vi "CANOpen_Main_Create and Send SDOs.vi"(7 "SDO Asynch":T1 {"HW Dyn Read"."Resp Chan."."Chan Refs" format="%.0x"; "HW Dyn Read"."Req Chan."."Chan Refs" format="%.0x"; "HW Dyn Write"."Resp Chan."."Chan Refs" format="%.0x"; "HW Dyn Write"."Req Chan."."Chan Refs" format="%.0x"; "List SDO"."Resp Chan."."Chan Refs" format="%.0x"; "List SDO"."Req Chan."."Chan Refs" format="%.0x"}, 8 "error in (no error)":errorcluster, 9 "Node States":u16[](array[ring]) items=["unknown"=1, "bootup"=0, "stopped"=4, "operational"=5, "pre-operational"=127, "connection lost"=128], 10 "Nodes":T3[](array[typedef]) {"NMT"."Node init static SDO state" items=["start remote node"=1, "enter pre-operational"=128]; "NMT"."Node run state" items=["start remote node"=1, "stop remote node"=2, "enter pre-operational"=128, "reset node"=129, "reset communication"=130]; "Dynamic SDOs"."Sub-Index (0)" format="%.0x"; "Dynamic SDOs"."Object Index" format="%.0x"; "Dynamic SDOs"."Block Data" format="%.0x"; "RPDOs"."PDO Channel" items=["PDO 1", "PDO 2", "PDO 3", "PDO 4"]; "RPDOs"."Parameters"."Bit Offset" max=8 step=1; "RPDOs"."Parameters"."Byte Offset" max=8 step=1; "TPDOs"."PDO Channel" items=["PDO 1", "PDO 2", "PDO 3", "PDO 4"]; "TPDOs"."Parameters"."Bit Offset" max=8 step=1; "TPDOs"."Parameters"."Byte Offset" max=8 step=1; "SDOs"."Sub-Index (0)" format="%.0x"; "SDOs"."Object Index" format="%.0x"; "SDOs"."Block Data" format="%.0x"}, 11 "interface object":refnum<k20>) -> (0 "error out":errorcluster, 3 "interface object out":refnum<k20>)   [LabVIEW 2013]
uses:
  SubVIS/CANOpen_Node Message Settings.ctl
  Shared Code/CANOpen_PDO Settings.ctl
  Shared Code/CANOpen_PDO Parameter Settings.ctl
  Shared Code/CANOpen_PDO Data Type.ctl
  System Explorer/SubVIs/CANopen Byte Order.ctl
  Shared Code/CANOpen_SDO Settings.ctl
  SubVIS/CANOpen_NMT Settings.ctl
  CanOpen_NMT_Config.ctl
  CanOpen_NMT_Static detect.ctl
  SubVIS/CANOpen_VS SDOs Data Refs.ctl
  <vilib>/NI Veristand/Custom Device API/Data Reference.ctl
  CanOpen_SDO Dynamic queue.ctl
  Shared Code/CANOpen_SDO queue W data.ctl
  Shared Code/CANOpen_SDO queue mode.ctl
  Shared Code/CANOpen_PDO Data Type in queue.ctl
  <vilib>/CANopenLib/CANOPEN.llb/CANopen SDO Create.vi
  <vilib>/CANopenLib/CANOPEN.llb/CANopen SDO Write [Block].vi
  <vilib>/CANopenLib/CANOPEN.llb/CANopen SDO Close.vi
  CANOpen Addon Custom Device.lvlib
  <vilib>/NI Veristand/Custom Device API/Custom Device API.lvlib
panel:
  # "LSB"
  # "MSB"
  # "LSB"
  # "MSB"
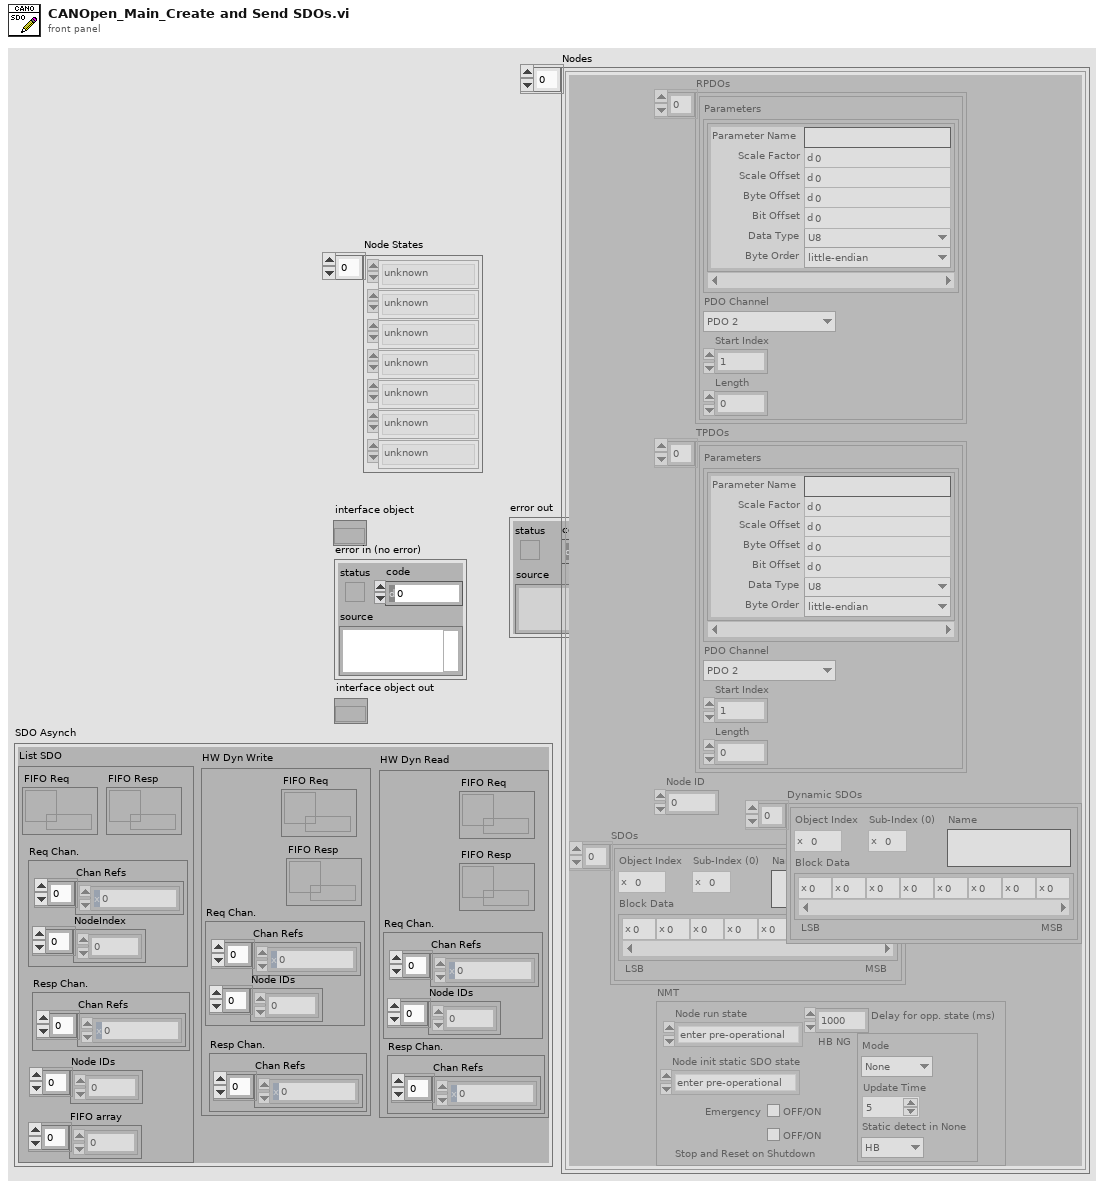
[diagram p1: front panel]
types:
  T1 = typedef "CANOpen Addon Custom Device.lvlib/CANOpen_VS SDOs Data Refs.ctl" = cluster{"List SDO":cluster{"FIFO Req":refnum<k33>, "Req Chan.":cluster{"Chan Refs":T2[], "NodeIndex":dbl[]}, "FIFO Resp":refnum<k33>, "Resp Chan.":cluster{"Chan Refs":T2[]}, "Node IDs":u8[], "FIFO array":dbl[]}, "HW Dyn Write":cluster{"FIFO Req":refnum<k33>, "FIFO Resp":refnum<k33>, "Req Chan.":cluster{"Chan Refs":T2[], "Node IDs":u8[]}, "Resp Chan.":cluster{"Chan Refs":T2[]}}, "HW Dyn Read":cluster{"FIFO Req":refnum<k33>, "FIFO Resp":refnum<k33>, "Req Chan.":cluster{"Chan Refs":T2[], "Node IDs":u8[]}, "Resp Chan.":cluster{"Chan Refs":T2[]}}}
  T2 = typedef "Custom Device API.lvlib/Data Reference.ctl" = i32
  T3 = typedef "CANOpen_Node Message Settings.ctl" = cluster{"RPDOs":T4[], "TPDOs":T4[], "Node ID":u8, "SDOs":T8[], "Dynamic SDOs":T8[], "NMT":T9}
  T4 = typedef "CANOpen Addon Custom Device.lvlib/CANOpen_PDO Settings.ctl" = cluster{"Parameters":T5[], "PDO Channel":u8, "Start Index":u32, "Length":u32}
  T5 = typedef "CANOpen Addon Custom Device.lvlib/CANOpen_PDO Parameter Settings.ctl" = cluster{"Parameter Name":string, "Scale Factor":dbl, "Scale Offset":dbl, "Byte Offset":u8, "Bit Offset":u8, "Data Type":T6, "Byte Order":T7}
  T6 = typedef "CANOpen Addon Custom Device.lvlib/CANOpen_PDO Data Type.ctl" = enum16{"U8", "U16", "U32", "I8", "I16", "I32", "Single", "Double", "Boolean"}
  T7 = typedef "CANOpen Addon Custom Device.lvlib/CANopen Byte Order.ctl" = enum16{"big-endian network order", "little-endian"}
  T8 = typedef "CANOpen Addon Custom Device.lvlib/CANOpen_SDO Settings.ctl" = cluster{"Object Index":u16, "Sub-Index (0)":u8, "Block Data":u8[], "Name":string}
  T9 = typedef "CANOpen Addon Custom Device.lvlib/CANOpen_NMT Settings.ctl" = cluster{"Node run state":u16, "Emergency":bool, "HB NG":T10, "Delay for opp. state (ms)":dbl, "Node init static SDO state":u16, "Stop and Reset on Shutdown":bool}
  T10 = typedef "CANOpen Addon Custom Device.lvlib/CanOpen_NMT_Config.ctl" = cluster{"Mode":T11, "Update Time":u16, "Static detect in None":T11}
  T11 = typedef "CANOpen Addon Custom Device.lvlib/CanOpen_NMT_Static detect.ctl" = enum16{"None", "HB", "NG"}
  T12 = typedef "CANOpen Addon Custom Device.lvlib/CANOpen_SDO queue mode.ctl" = enum16{"WRITE write", "WRITE response", "READ write", "READ response"}
  T13 = typedef "CANOpen Addon Custom Device.lvlib/CANOpen_PDO Data Type in queue.ctl" = enum16{"U8", "U16", "U32", "I8", "I16", "I32", "Single", "Double"}
  T14 = typedef "CANOpen Addon Custom Device.lvlib/CanOpen_SDO Dynamic queue.ctl" = cluster{"Node ID":u8, "Data":T15}
  T15 = typedef "CANOpen Addon Custom Device.lvlib/CANOpen_SDO queue W data.ctl" = cluster{"Object Index":u16, "Object Sub-Index (0)":u8, "Mode":T12, "Data Type":T13, "Value":dbl, "Status code":dbl, "Byte Order":enum16{"big-endian, network order", "little-endian"}}
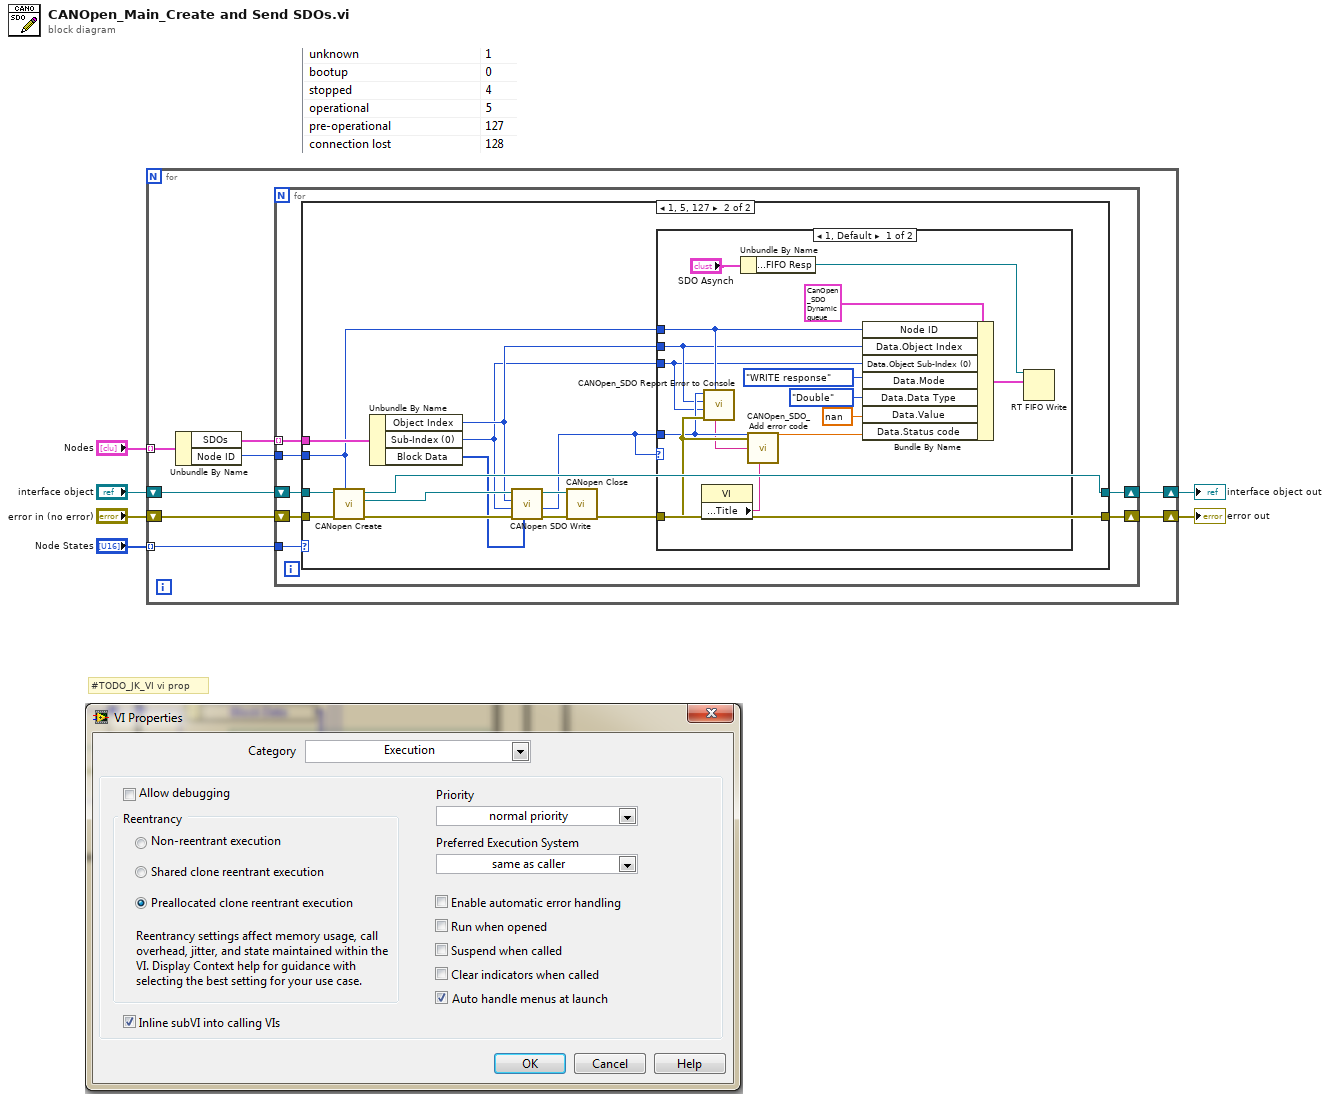
[diagram p0: block diagram]
diagram:
  # "#TODO_JK_VI vi prop"
  n1 = for {
    shift-right: [w11] -> w3
    shift-left: "interface object" -> [w12]
    shift-right: [w13] -> w2
    shift-left: "error in (no error)" -> [w14]
    tunnel: "Nodes" -> [w10] mode=indexing
    tunnel: "Node States" -> [w7] mode=indexing
    n2 = Unbundle By Name(w10) -> ("SDOs"=w8:T8[], "Node ID"=w9:u8)
    n3 = for {
      tunnel: w9 -> [w17]
      shift-right: [w18] -> w11
      shift-left: w12 -> [w19]
      shift-right: [w20] -> w13
      shift-left: w14 -> [w21]
      tunnel: w8 -> [w16] mode=indexing
      tunnel: w7 -> [w15]
      n4 = case shown="1, 5, 127" w15 {
        tunnel: w21 -> [w22 w34]
        tunnel: [w22 w28] -> w20
        tunnel: w19 -> [w23 w32]
        tunnel: [w23 w31] -> w18
        tunnel: w17 -> [_ w27]
        tunnel: w16 -> [_ w30]
        frame 0, Default {
        }
        frame 1, 5, 127 {
          n5 = call-poly <vilib>:"CANopen Create.vi"("node-ID"=w27, "error in (no error)"=w34, "interface object in"=w32) -> ("error out"=w36:errorcluster, "SDO object out"=w37:refnum<k20>, "interface object out"=w31:refnum<k20>)  [unwired: 6 in]
          n6 = Unbundle By Name(w30) -> ("Object Index"=w26:u16, "Sub-Index (0)"=w25:u8, "Block Data"=w29:u8[])
          n7 = call-poly <vilib>:"CANopen SDO Write.vi"("block data"=w29, "error in (no error)"=w36, "object sub-index (0)"=w25, "object index"=w26, "SDO object in"=w37) -> ("error out"=w35:errorcluster, "completion code"=w24:u32, "SDO object out"=w33:refnum<k20>)  [unwired: 4 in]
          n8 = call-poly <vilib>:"CANopen Close.vi"("error in (no error)"=w35, "SDO object in"=w33) -> ("error out"=w28:errorcluster)  [unwired: 9 in]
          n9 = case shown="1, Default" w24 {
            tunnel: w24 -> [w43 _]
            tunnel: w28 -> [w45 _]
            tunnel: w27 -> [w44 _]
            tunnel: w26 -> [w40 _]
            tunnel: w25 -> [w39 _]
            frame 1, Default {
              n10 = property class="VI"() -> ("Front Panel.Title"=w38:string)  [unwired: 2 in, 2 out]
              n11 = call "CANOpen_SDO Report Error to Console.vi"("Caller"=w38, "Node ID"=w44, "error in (no error)"=w45, "Object Sub-Index"=w39, "Object Index"=w40, "completion code"=w43) -> ()  [unwired: 6 in]
              n12 = Unbundle By Name("SDO Asynch") -> ("HW Dyn Write.FIFO Resp"=w41:refnum<k33>)
              n13 = call "CANOpen_SDO_Add error code.vi"("completion code in"=w43, "error in (no error)"=w45) -> ("completion code out"=w46:dbl)  [unwired: 25 in]
              n14 = Bundle By Name(cluster=T14 {"Node ID"=0, "Data"={"Object Index"=0, "Object Sub-Index (0)"=0, "Mode"=enum."WRITE response", "Data Type"=enum."Double", "Value"=0.0, "Status code"=0.0, "Byte Order"=enum."big-endian, network order"}} ("element"), "Node ID"=w44, "Data.Object Index"=w40, "Data.Object Sub-Index (0)"=w39, "Data.Mode"=CANOpen_SDO_queue_mode."WRITE response", "Data.Data Type"=CANOpen_PDO_Data_Type_in_queue."Double", "Data.Value"=nan, "Data.Status code"=w46) -> (w48:T14)
              n15 = RT FIFO Write(0:w41, 1:w48) -> ()  [unwired: 3 in, 4 out]
            }
            frame 0 {
            }
          }
        }
      }
    }
  }
  "error out" <- w2
  "interface object out" <- w3
